vi "Read UNSUBSCRIBE Request Data (JSON).vi"(8 "error in (no error)":errorcluster, 11 "Unsubscribe JSON in":refnum<class "Unsubscribe JSON.lvclass">) -> (0 "error out":errorcluster, 2 "UNSUBSCRIBE Request Data (JSON).ctl":T1, 3 "Unsubscribe JSON out":refnum<class "Unsubscribe JSON.lvclass">)   [LabVIEW 2020, in "wamplv.lvlib" / "Unsubscribe JSON.lvclass"]
uses:
  Unsubscribe JSON.lvclass
  WAMP Client/Private/TypeDef/UNSUBSCRIBE Request Data (JSON).ctl
  Unsubscribe JSON.lvclass/Unsubscribe JSON.ctl
  wamplv.lvlib
  Message loop classes/ErrorOrSuccess JSON/ErrorOrSuccess JSON.lvclass
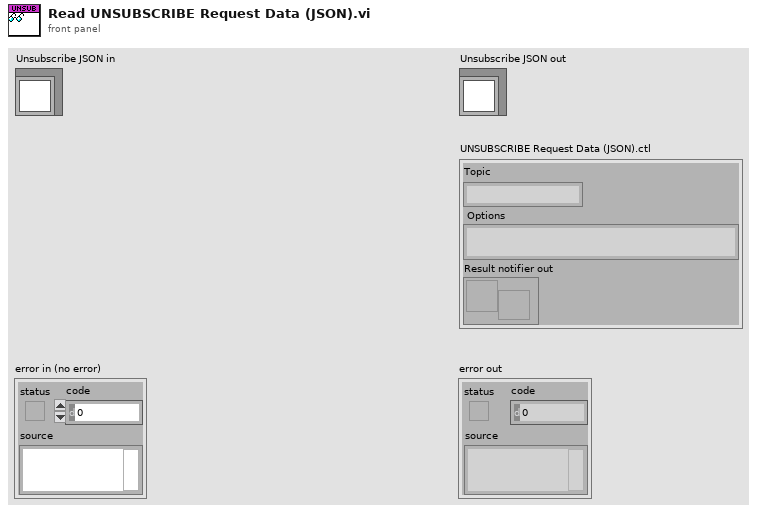
[diagram p1: front panel]
types:
  T1 = typedef "wamplv.lvlib/UNSUBSCRIBE Request Data (JSON).ctl" = cluster{"Topic":string, "Options":string, "Result notifier out":refnum<notifier>}
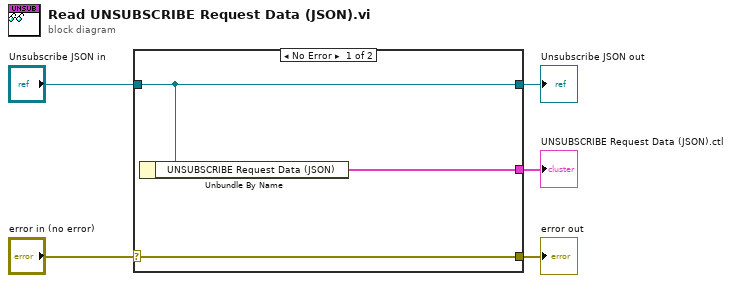
[diagram p0: block diagram]
diagram:
  n1 = case shown="No Error" "error in (no error)" {
    selector: "error in (no error)" -> [w8 w9]
    tunnel: [w8 w9] -> w4
    tunnel: [w7 w10] -> w2
    tunnel: "Unsubscribe JSON in" -> [w7 w10]
    tunnel: [w6 _] -> w1
    frame No Error {
      n2 = Unbundle By Name(w7) -> ("UNSUBSCRIBE Request Data (JSON)"=w6:T1)
    }
    frame Error {
    }
  }
  "error out" <- w4
  "Unsubscribe JSON out" <- w2
  "UNSUBSCRIBE Request Data (JSON).ctl" <- w1
